vi "onListTestCases.vi"(8 "error in (no error)":errorcluster, 10 "Filter":T1, 11 "Pips.TestResults in":refnum<class "Pips.TestResults.lvclass">) -> (0 "error out":errorcluster, 2 "TestCases":string[](array[string]), 3 "Pips.TestResults out":refnum<class "Pips.TestResults.lvclass">)   [LabVIEW 2021, in "Banana.Caraya.lvlib" / "Pips.TestResults.lvclass"]
uses:
  Pips.TestResults.lvclass
  Pips.TestResults.lvclass/Pips.TestResults.ctl
  1ce79d66-3172-4516-944e-74ae46fd5f68.vi
  810e7706-8876-46fe-9905-bab50fed7d99.vi
  Bananas/Pips/pip_filter -- enum.ctl
  Bananas/Pips/Pips.lvclass
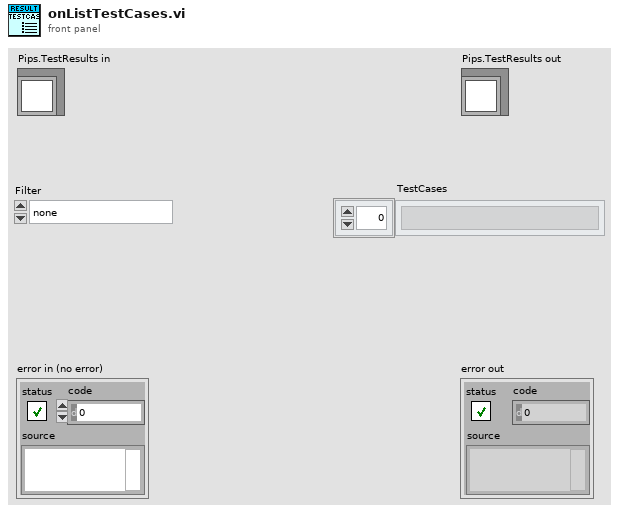
[diagram p1: front panel]
types:
  T1 = typedef "Bananas.lvlib/Pips.lvclass/pip_filter -- enum.ctl" = enum16{"none", "passed", "skipped", "covered", "uncovered"}
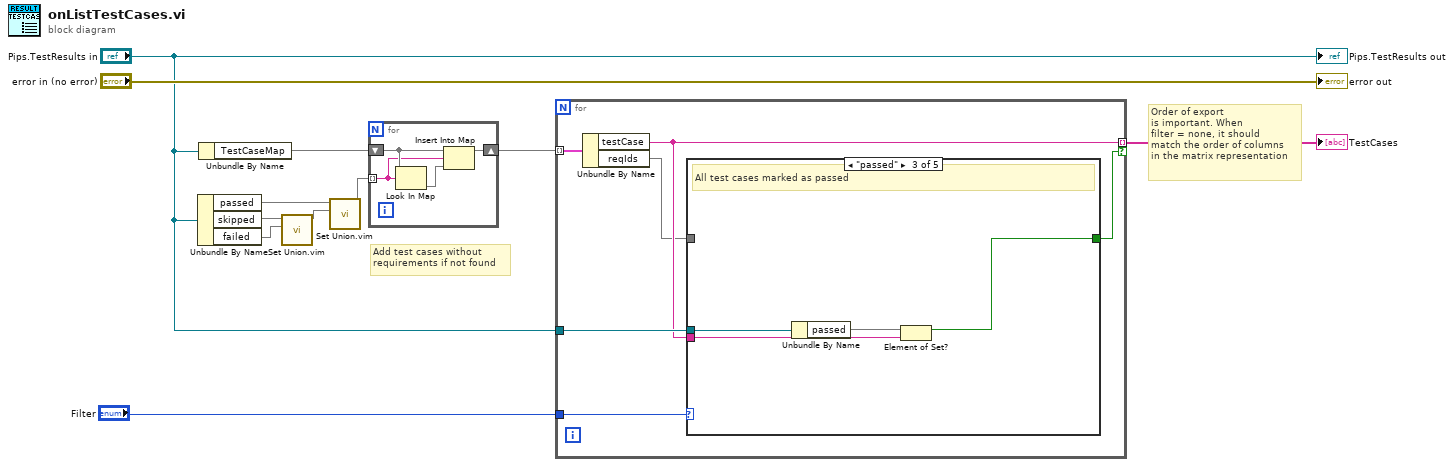
[diagram p0: block diagram]
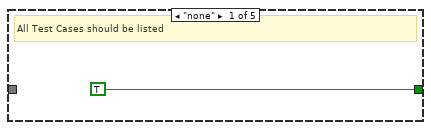
[diagram p2: hidden frame]
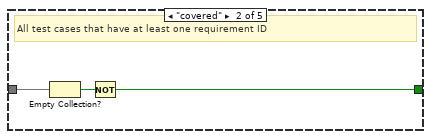
[diagram p3: hidden frame]
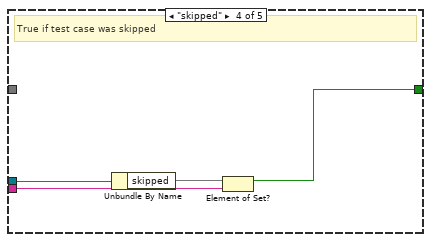
[diagram p4: hidden frame]
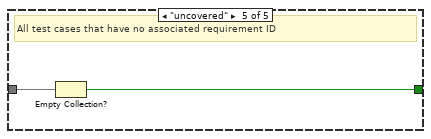
[diagram p5: hidden frame]
diagram:
  # "Add test cases without\nrequirements if not found"
  # "Order of export\nis important. When\nfilter = none, it should\nmatch the order of columns\nin the matrix representation"
  n1 = Unbundle By Name("Pips.TestResults in") -> ("passed"=w8:set{string}, "skipped"=w7:set{string}, "failed"=w6:set{string})
  n2 = Unbundle By Name("Pips.TestResults in") -> ("TestCaseMap"=w4:map{string, set{string}})
  n3 = call "Set Union.vim"("set 2"=w6, "set 1"=w7) -> ("union"=w5:set{string})  [unwired: 9 in]
  n4 = call "Set Union.vim"("set 2"=w5, "set 1"=w8) -> ("union"=w2:set{string})  [unwired: 9 in]
  n5 = for {
    shift-right: [w12] -> w3
    shift-left: w4 -> [w15]
    tunnel: w2 -> [w13] mode=indexing
    n6 = Look In Map(map=w15, key=w13) -> (value=w14:set{string})  [unwired: 1 in, 1 out]
    n7 = Insert Into Map(map in=w15, key=w13, value=w14) -> (map out=w12:map{string, set{string}})  [unwired: 2 out]
  }
  n8 = for {
    tunnel: w3 -> [w21] mode=indexing
    tunnel: [w17] -> w10 mode=indexing if=w19
    tunnel: "Filter" -> [w20]
    tunnel: "Pips.TestResults in" -> [w18]
    n9 = Unbundle By Name(w21) -> ("testCase"=w17:string, "reqIds"=w16:set{string})
    n10 = case shown="\"passed\"" w20 {
      tunnel: w16 -> [_ w25 _ _ w35]
      tunnel: [TRUE w23 w26 w30 w34] -> w19
      tunnel: w18 -> [_ _ w29 w33 _]
      tunnel: w17 -> [_ _ w27 w31 _]
      frame "none" {
        # "All Test Cases should be listed"
      }
      frame "covered" {
        # "All test cases that have at least one requirement ID"
        n11 = Empty Collection?(1:w25) -> (0:w24:bool)
        n12 = Not(x=w24) -> (.not. x?=w23:bool)
      }
      frame "passed" {
        # "All test cases marked as passed"
        n13 = Unbundle By Name(w29) -> ("passed"=w28:set{string})
        n14 = Element of Set?(10:w27, 11:w28) -> (3:w26:bool)
      }
      frame "skipped" {
        # "True if test case was skipped"
        n15 = Unbundle By Name(w33) -> ("skipped"=w32:set{string})
        n16 = Element of Set?(10:w31, 11:w32) -> (3:w30:bool)
      }
      frame "uncovered" {
        # "All test cases that have no associated requirement ID"
        n17 = Empty Collection?(1:w35) -> (0:w34:bool)
      }
    }
  }
  "TestCases" <- w10
  "error out" <- "error in (no error)"
  "Pips.TestResults out" <- "Pips.TestResults in"
